vi "(백업)ATC예문V2.vi"() -> ()   [LabVIEW 2014]
doc: "ATC app"
uses:
  <vilib>/Utility/sysdir.llb/System Directory Type.ctl
panel:
  in  "정규식 5":string
  in  "정규식 4":string
  in  "?":bool
  in  "?":bool
  in  "정규식 3":string
  out "ip address":string="ip address"
  in  "탭":T1(tab)
  in  "도움말":bool
  in  "메모":string="필요한 메모를 할수 있습니다. "
  in  "SID&RadarVector. 2":string="SID&RadarVector. "
  in  "인사말":string="인사말"
  in  "관제기관":string="관제기관"
  in  "콜사인":string="콜사인\n콜사인\n콜사인"
  in  "도착공항":string="도착공항"
  in  "SID&RadarVector":string="SID&RadarVector"
  in  "비행고도":string="비행고도"
  in  "인사말2":string="인사말"
  in  "콜사인2":string="콜사인"
  in  "콜사인3":string="콜사인"
  in  "콜사인4":string="콜사인"
  in  "콜사인5":string="콜사인"
  in  "콜사인6":string="콜사인"
  in  "도착공항2":string="도착공항"
  in  "제한고도":string="제한고도"
  in  "비행고도2":string="비행고도"
  in  "D접속주파수":string="접속주파수"
  in  "스콱번호":string="스콱번호"
  in  "도착공항3":string="도착공항"
  in  "SID&RadarVector. 3":string="SID&RadarVector. "
  in  "제한고도2":string="제한고도"
  in  "비행고도3":string="비행고도"
  in  "D접속주파수2":string="접속주파수"
  in  "스콱번호2":string="스쾃번호"
  in  "콜사인7":string="콜사인"
  in  "콜사인8":string="콜사인"
  in  "관제기관":string="관제기관"
  in  "G접속주파수2":string="접속주파수"
  in  "관제기관":string="관제기관"
  in  "G접속주파수":string="접속주파수"
  in  "콜사인9":string="콜사인"
  in  "정보1":bool
  in  "도움말 2":bool
  in  "유도로 2":string="유도로"
  in  "유도로":string="유도로"
  in  "방향 2":string="방향"
  in  "방향":string="방향"
  in  "메모2":string="필요한 메모를 할수 있습니다. "
  in  "관제기관":string="관제기관"
  in  "콜사인24":string="콜사인"
  in  "T접속주파수2":string="접속주파수"
  in  "T접속주파수":string="접속주파수"
  in  "관제기관8":string="관제기관"
  in  "콜사인23":string="콜사인"
  in  "활주로9":string="활주로"
  in  "관제기관7":string="관제기관"
  in  "콜사인22":string="콜사인"
  in  "콜사인21":string="콜사인"
  in  "콜사인20":string="콜사인"
  in  "콜사인19":string="콜사인"
  in  "활주로8":string="활주로"
  in  "활주로7":string="활주로"
  in  "콜사인17":string="콜사인"
  in  "활주로6":string="활주로"
  in  "콜사인18":string="콜사인"
  in  "활주로5":string="활주로"
  in  "콜사인16":string="콜사인"
  in  "활주로4":string="활주로"
  in  "콜사인15":string="콜사인"
  in  "활주로3":string="활주로"
  in  "콜사인14":string="콜사인"
  in  "콜사인13":string="콜사인"
  in  "현재기압2":string="현재기압"
  in  "출발공항":string="출발공항"
  in  "활주로2":string="활주로"
  in  "현재기압":string="현재기압"
  in  "출발공항2":string="출발공항"
  in  "활주로1":string="활주로"
  in  "콜사인12":string="콜사인"
  in  "콜사인11":string="콜사인"
  in  "관제기관":string="관제기관"
  in  "인사3":string="인사"
  in  "정보2":bool
  in  "도움말 3":bool
  in  "콜사인34 2":string="콜사인"
  in  "관제기관 2":string="관제기관"
  in  "관제기관":string="관제기관"
  in  "관제기관":string="관제기관"
  in  "메모3":string="필요한 메모를 할수 있습니다. "
  in  "인사4":string="인사"
  in  "콜사인25":string="콜사인"
  in  "활주로10":string="활주로"
  in  "콜사인26":string="콜사인"
  in  "바람방향":string="바람방향"
  in  "풍속":string="풍속"
  in  "콜사인28":string="콜사인"
  in  "활주로13":string="활주로"
  in  "콜사인29":string="콜사인"
  in  "활주로12":string="활주로"
  in  "콜사인30":string="콜사인"
  in  "활주로14":string="활주로"
  in  "콜사인31":string="콜사인"
  in  "활주로15":string="활주로"
  in  "관제기관":string="관제기관"
  in  "콜사인32":string="콜사인"
  in  "현재고도":string="현재고도"
  in  "허가고도":string="허가고도"
  in  "콜사인33":string="콜사인"
  in  "접속주파수":string="접속주파수"
  in  "콜사인34":string="콜사인"
  in  "접속주파수2":string="접속주파수"
  in  "정보3":bool
  in  "도움말 4":bool
  in  "순항고도or이니셜고도":string="순항고도or이니셜고도"
  in  "관제기관 3":string="관제기관"
  in  "메모 4":string="필요한 메모를 할수 있습니다. "
  in  "인사5":string="인사"
  in  "관제기관":string="관제기관"
  in  "콜사인35":string="콜사인"
  in  "현재고도A":string="현재고도"
  in  "콜사인36":string="콜사인"
  in  "관제기관":string="관제기관"
  in  "허가고도4":string="허가고도"
  in  "허가고도5":string="허가고도"
  in  "콜사인37":string="콜사인"
  in  "콜사인38":string="콜사인"
  in  "허가고도6":string="허가고도"
  in  "허가고도7":string="허가고도"
  in  "콜사인39":string="콜사인"
  in  "콜사인40":string="콜사인"
  in  "관제기관":string="관제기관"
  in  "A접속주파수":string="접속주파수"
  in  "관제기관14":string="관제기관"
  in  "A접속주파수2":string="접속주파수"
  in  "콜사인41":string="콜사인"
  in  "정보4":bool
  in  "콜사인38 2":string="콜사인"
  in  "관제기관 4":string="관제기관"
  in  "허가고도6 2":string="허가고도"
  in  "허가고도6 3":string="허가고도"
  in  "콜사인39 2":string="콜사인"
  in  "메모5":string="필요한 메모를 할수 있습니다. "
  in  "도움말 5":bool
  in  "정보5":bool
  in  "인사말 2":string="인사말"
  in  "허가고도 2":string="허가고도"
  in  "지점":string="지점"
  in  "허가고도7 2":string="허가고도"
  in  "콜사인38 3":string="콜사인"
  in  "콜사인39 3":string="콜사인"
  in  "허가고도7 3":string="허가고도"
  in  "지점 2":string="지점"
  in  "메모6":string="필요한 메모를 할수 있습니다. "
  in  "도움말 6":bool
  in  "관제기관":string="관제기관"
  in  "콜사인46":string="콜사인"
  in  "날시정보":string="날시정보"
  in  "고도":string="고도"
  in  "콜사인47":string="콜사인"
  in  "관제기관":string="관제기관"
  in  "L활주로":string="활주로"
  in  "도착공항4":string="도착공항"
  in  "현재기압":string="현재기압"
  in  "콜사인48":string="콜사인"
  in  "관제기관5":string="관제기관"
  in  "L활주로":string="활주로"
  in  "도착공항5":string="도착공항"
  in  "현재기압":string="현재기압"
  in  "콜사인49":string="콜사인"
  in  "고도":string="고도"
  in  "콜사인50":string="콜사인"
  in  "고도":string="고도"
  in  "콜사인51":string="콜사인"
  in  "고도":string="고도"
  in  "고도":string="고도"
  in  "콜사인52":string="콜사인"
  in  "콜사인53":string="콜사인"
  in  "관제기관":string="관제기관"
  in  "풍속":string="풍속"
  in  "바람방향":string="바람방향"
  in  "L활주로3":string="활주로"
  in  "콜사인54":string="콜사인"
  in  "L활주로":string="활주로"
  in  "콜사인55":string="콜사인"
  in  "관제기관":string="관제기관"
  in  "L활주로":string="활주로"
  in  "ILS":string="주파수(ils)"
  in  "콜사인56":string="콜사인"
  in  "L활주로6":string="활주로"
  in  "ILS2":string="주파수(ils)"
  in  "콜사인57":string="콜사인"
  in  "T관제기관":string="관제기관"
  in  "T접속주파수":string="접속주파수"
  in  "콜사인58":string="콜사인"
  in  "콜사인59":string="콜사인"
  in  "관제기관":string="관제기관"
  in  "T접속주파수":string="접속주파수"
  in  "정보6":bool
  in  "메모7":string="필요한 메모를 할수 있습니다. "
  in  "도움말 7":bool
  in  "바람방향":string="바람방향"
  in  "관제기관":string="관제기관"
  in  "콜사인60":string="콜사인"
  in  "L활주로7":string="활주로"
  in  "콜사인61":string="콜사인"
  in  "풍속":string="풍속"
  in  "콜사인62":string="콜사인"
  in  "L활주로":string="활주로"
  in  "L활주로":string="활주로"
  in  "관제기관":string="관제기관"
  in  "콜사인63":string="콜사인"
  in  "관제기관3":string="관제기관"
  in  "콜사인64":string="콜사인"
  in  "L활주로":string="활주로"
  in  "G관제기관":string="관제기관"
  in  "G접속주파수":string="접속주파수"
  in  "콜사인65":string="콜사인"
  in  "관제기관":string="관제기관"
  in  "G접속주파수":string="접속주파수"
  in  "정보7":bool
  in  "콜사인70":string="콜사인"
  in  "C활주로3":string="활주로"
  in  "C활주로2":string="활주로"
  in  "관제기관3 2":string="관제기관"
  in  "C활주로":string="활주로"
  in  "콜사인69":string="콜사인"
  in  "관제기관2":string="관제기관"
  in  "메모8":string="필요한 메모를 할수 있습니다. "
  in  "도움말 8":bool
  in  "관제기관":string="관제기관"
  in  "콜사인66":string="콜사인"
  in  "콜사인67":string="콜사인"
  in  "게이트번호":string="게이트번호"
  in  "THEN":string="then"
  in  "콜사인68":string="콜사인"
  in  "게이트번호2":string="게이트번호"
  in  "THEN2":string="then"
  in  "콜사인10":string="콜사인"
  in  "관제기관4":string="관제기관"
  in  "콜사인71":string="콜사인"
  in  "콜사인72":string="콜사인"
  in  "정보8":bool
  # "ver.Beta.2.2.0"
  # "~"
  # "Good"
  # "Clearance Delivery"
  # "Pilot"
  # "at FL"
  # "Request IFR Clearance to"
  # "Airport via"
  # "~"
  # "Good"
  # "Controller"
  # ",  Clearance  Delivery, standby."
  # "Pilot"
  # "Stand by,"
  # "Controller"
  # "Delivery 또는 Delivery, Are you ready to copy?"
  # "Pilot"
  # "Go Ahead 또는 Ready to copy"
  # "Airport via"
  # ", Cleared to"
  # "Controller"
  # "ft expect FL"
  # "then as filed. Climb and Maintain"
  # "Departure Frequency"
  # "Read back."
  # "Squawk"
  # "Pilot"
  # "Airport via"
  # "Cleared to"
  # ","
  # "then as filed."
  # "Climb and Maintain"
  # "ft expect FL"
  # "Departure Frequency"
  # "and  Squawk"
  # "Controller"
  # ", Read back is corrent contact"
  # "Ground"
  # "bye bye~."
  # "Pilot"
  # "Roger, contact"
  # ", bye bye~"
  # "ver.Beta.2.2.0"
  # "Pilot"
  # "~"
  # "Good"
  # "ready for push back and Engine Start."
  # ","
  # ", Rwy"
  # "Push Back and Engine Start Approved, heading to"
  # "Controller"
  # ","
  # "QNH"
  # "Read Back."
  # "Pilot"
  # "Roger\nPush Back and Engine Start Approved, heading to"
  # ", Rwy"
  # "QNH"
  # "Ready for taxi to the Rwy"
  # ","
  # "Pilot"
  # "- Push back 완료 후 -"
  # ", Ready for Taxi to Rwy"
  # "Controller"
  # ", taxi to"
  # "via taxiway"
  # ", Roger"
  # "Pilot"
  # "via taxiway"
  # "Taxi to"
  # "- 활주로를 건널 상황일 때 -"
  # "Pilot"
  # "Request Cross Rwy"
  # "Controller"
  # ", cleared Cross Rwy"
  # "Pilot"
  # "cleared Cross Rwy"
  # "Controller"
  # "Squawk Mode C."
  # "Pilot"
  # ", Roger squawk mode 'C'"
  # "------------------------ 홀딩 포인트 도착 후 ----------------------------------"
  # "hold short of Rwy"
  # ","
  # "Controller"
  # "Roger,"
  # "contact"
  # "Tower"
  # "bye bye~"
  # "Pilot"
  # "Contact"
  # "ver.Beta.2.2.0"
  # "Pilot"
  # "Good"
  # "~"
  # ",  hold short Rwy"
  # ", Ready for Departure"
  # "(곧바로 이륙허가)"
  # "Controller"
  # ", wind"
  # "knot, cleared for take off."
  # "at"
  # "(활주로 정렬대기)"
  # "Controller"
  # "Line up and wait Rwy"
  # "Pilot"
  # "Line up and wait Rwy"
  # "Roger,"
  # "(홀딩 포인트에서 대기)"
  # "Controller"
  # ", Hold short rwy"
  # ","
  # "Pilot"
  # "Hold short of Rwy"
  # "Roger,"
  # "- 이 륙 후 -"
  # "ft."
  # "Pilot"
  # "Airborn Passing"
  # "ft, Climbing"
  # ","
  # "Controller"
  # ", contact"
  # "Departure,"
  # "bye bye~"
  # "Pilot"
  # ", Roger"
  # "Contact"
  # "Departure,"
  # "bye bye~"
  # "ver.Beta.2.2.0"
  # "Good"
  # "~"
  # "Pilot"
  # "Passing"
  # "expect"
  # "with (SID)."
  # ","
  # ","
  # "Controller"
  # "Departure, Radar Contact, Climb via (SID) to"
  # ","
  # "."
  # "Pilot"
  # "Roger, Climb via"
  # ","
  # "-고도제한 해제시-"
  # "Controller"
  # "Departure, Radar Contact, Climb via (SID) to"
  # ", Cancel Level Restrictions."
  # "Pilot"
  # "Roger, Climb via (SID) to"
  # ", Cancel Level Restrictions,"
  # "-속도제한 해제시-"
  # "Controller"
  # "Departure, Radar Contact, Climb via (SID) to"
  # ", Cancel Speed Restrictions."
  # "Pilot"
  # "Roger, Climb via (SID) to"
  # ", Cancel Speed Restrictions,"
  # "Controller"
  # "Control,"
  # ", bye bye."
  # ", You are leaving my airspace, Contact"
  # "Pilot"
  # "Contact"
  # "G'day"
  # "Control,"
  # ","
  # "ver.Beta.2.2.0"
  # "Pilot"
  # "Good"
  # "Decend and maintain FL"
  # "with (SID)."
  # "-하강 발부-"
  # "Controller"
  # "by"
  # ", Descend and Maintain"
  # "Pilot"
  # "Descend and Maintain"
  # "by"
  # "Pilot"
  # "ver.Beta.2.2.0"
  # ","
  # "FL"
  # "with information"
  # ","
  # ", Expect vector to ILS Rwy"
  # "approach"
  # "Controller"
  # "QNH"
  # "Roger,"
  # "Pilot"
  # ", Expect vector to ILS Rwy"
  # "final approach"
  # "QNH"
  # "Controller"
  # ", Decend and maintain FL"
  # "Pilot"
  # "Decend and maintain FL"
  # "Roger,"
  # "Controller"
  # ", Decend and maintain"
  # "ft"
  # "Pilot"
  # "Roger"
  # "Decend and maintain"
  # "ft"
  # "Controller"
  # ","
  # "for landing"
  # "wind"
  # "knots active Rwy"
  # "at"
  # "Pilot"
  # "Roger,"
  # "Rwy"
  # "for landing"
  # "Controller"
  # ","
  # "approach use Rwy"
  # "ILS"
  # "Roger,"
  # "Pilot"
  # "Use Rwy"
  # "ILS"
  # "- 정 렬 후 -"
  # "Pilot"
  # "Approach,"
  # ", Established on Localizer."
  # "Controller"
  # "Tower,"
  # "Good day,"
  # "Roger, Contact"
  # "Pilot"
  # "Contact"
  # "Tower"
  # "Good day,"
  # "ver.Beta.2.2.0"
  # "Pilot"
  # ","
  # "Inbound Approaching Rwy"
  # "Controller"
  # ", Wind"
  # "at"
  # "knots Rwy"
  # ", Cleared to land"
  # "Pilot"
  # "Rwy"
  # "Cleared to land"
  # "Pilot"
  # ","
  # "- 착 륙 후 -"
  # ","
  # "Pilot"
  # "Touch down with Rwy"
  # "Controller"
  # "Roger, change squawk mode Standby and contact"
  # "bye bye~"
  # "ground"
  # "Pilot"
  # ", Roger"
  # "bye bye~"
  # "Change squawk mode standby and contact"
  # "- 활주로를 건널 상황일 때 -"
  # "Pilot"
  # ","
  # "Request Cross Rwy"
  # "Controller"
  # ", Cross Rwy"
  # "approved."
  # "Pilot"
  # "Cross Rwy"
  # "approved"
  # "ver.Beta.2.2.0"
  # ","
  # "Pilot"
  # "Ready to taxi to the Gate"
  # "Controller"
  # ", taxi to the gate"
  # "via taxi way"
  # "Roger,"
  # "Pilot"
  # "taxi to the gate"
  # "via taxi way"
  # "- 게이트 도착 후 -"
  # "Pilot"
  # "at Gate and Engine Shut down."
  # "Thank you for your ATC service."
  # "Controller"
  # ", at the gate and Engine Shut down, Thank you ~~"
  # "Pilot"
  # "Have a nice day,"
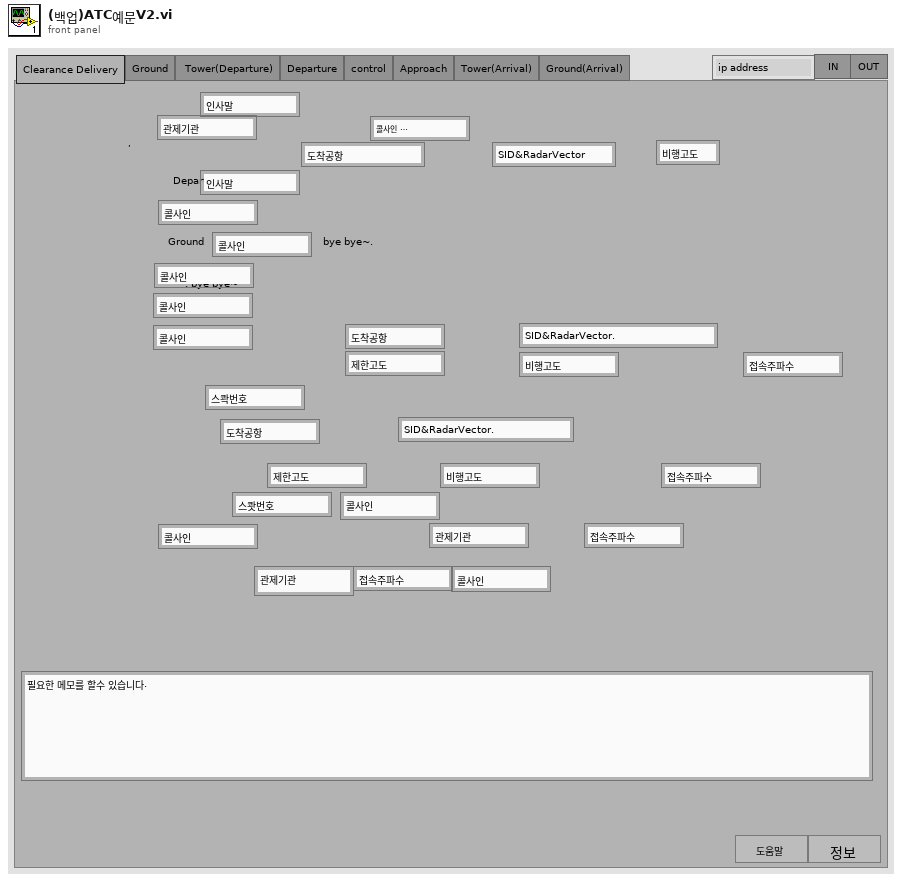
[diagram p1: front panel]
types:
  T1 = enum32{"Clearance Delivery", "Ground", " Tower(Departure)", "Departure", "control", "Approach", "Tower(Arrival)", "Ground(Arrival)"}
  T2 = enum16{"open", "replace", "create", "open or create", "replace or create", "replace or create with confirmation"}
  T3 = typedef "System Directory Type.ctl" = i32
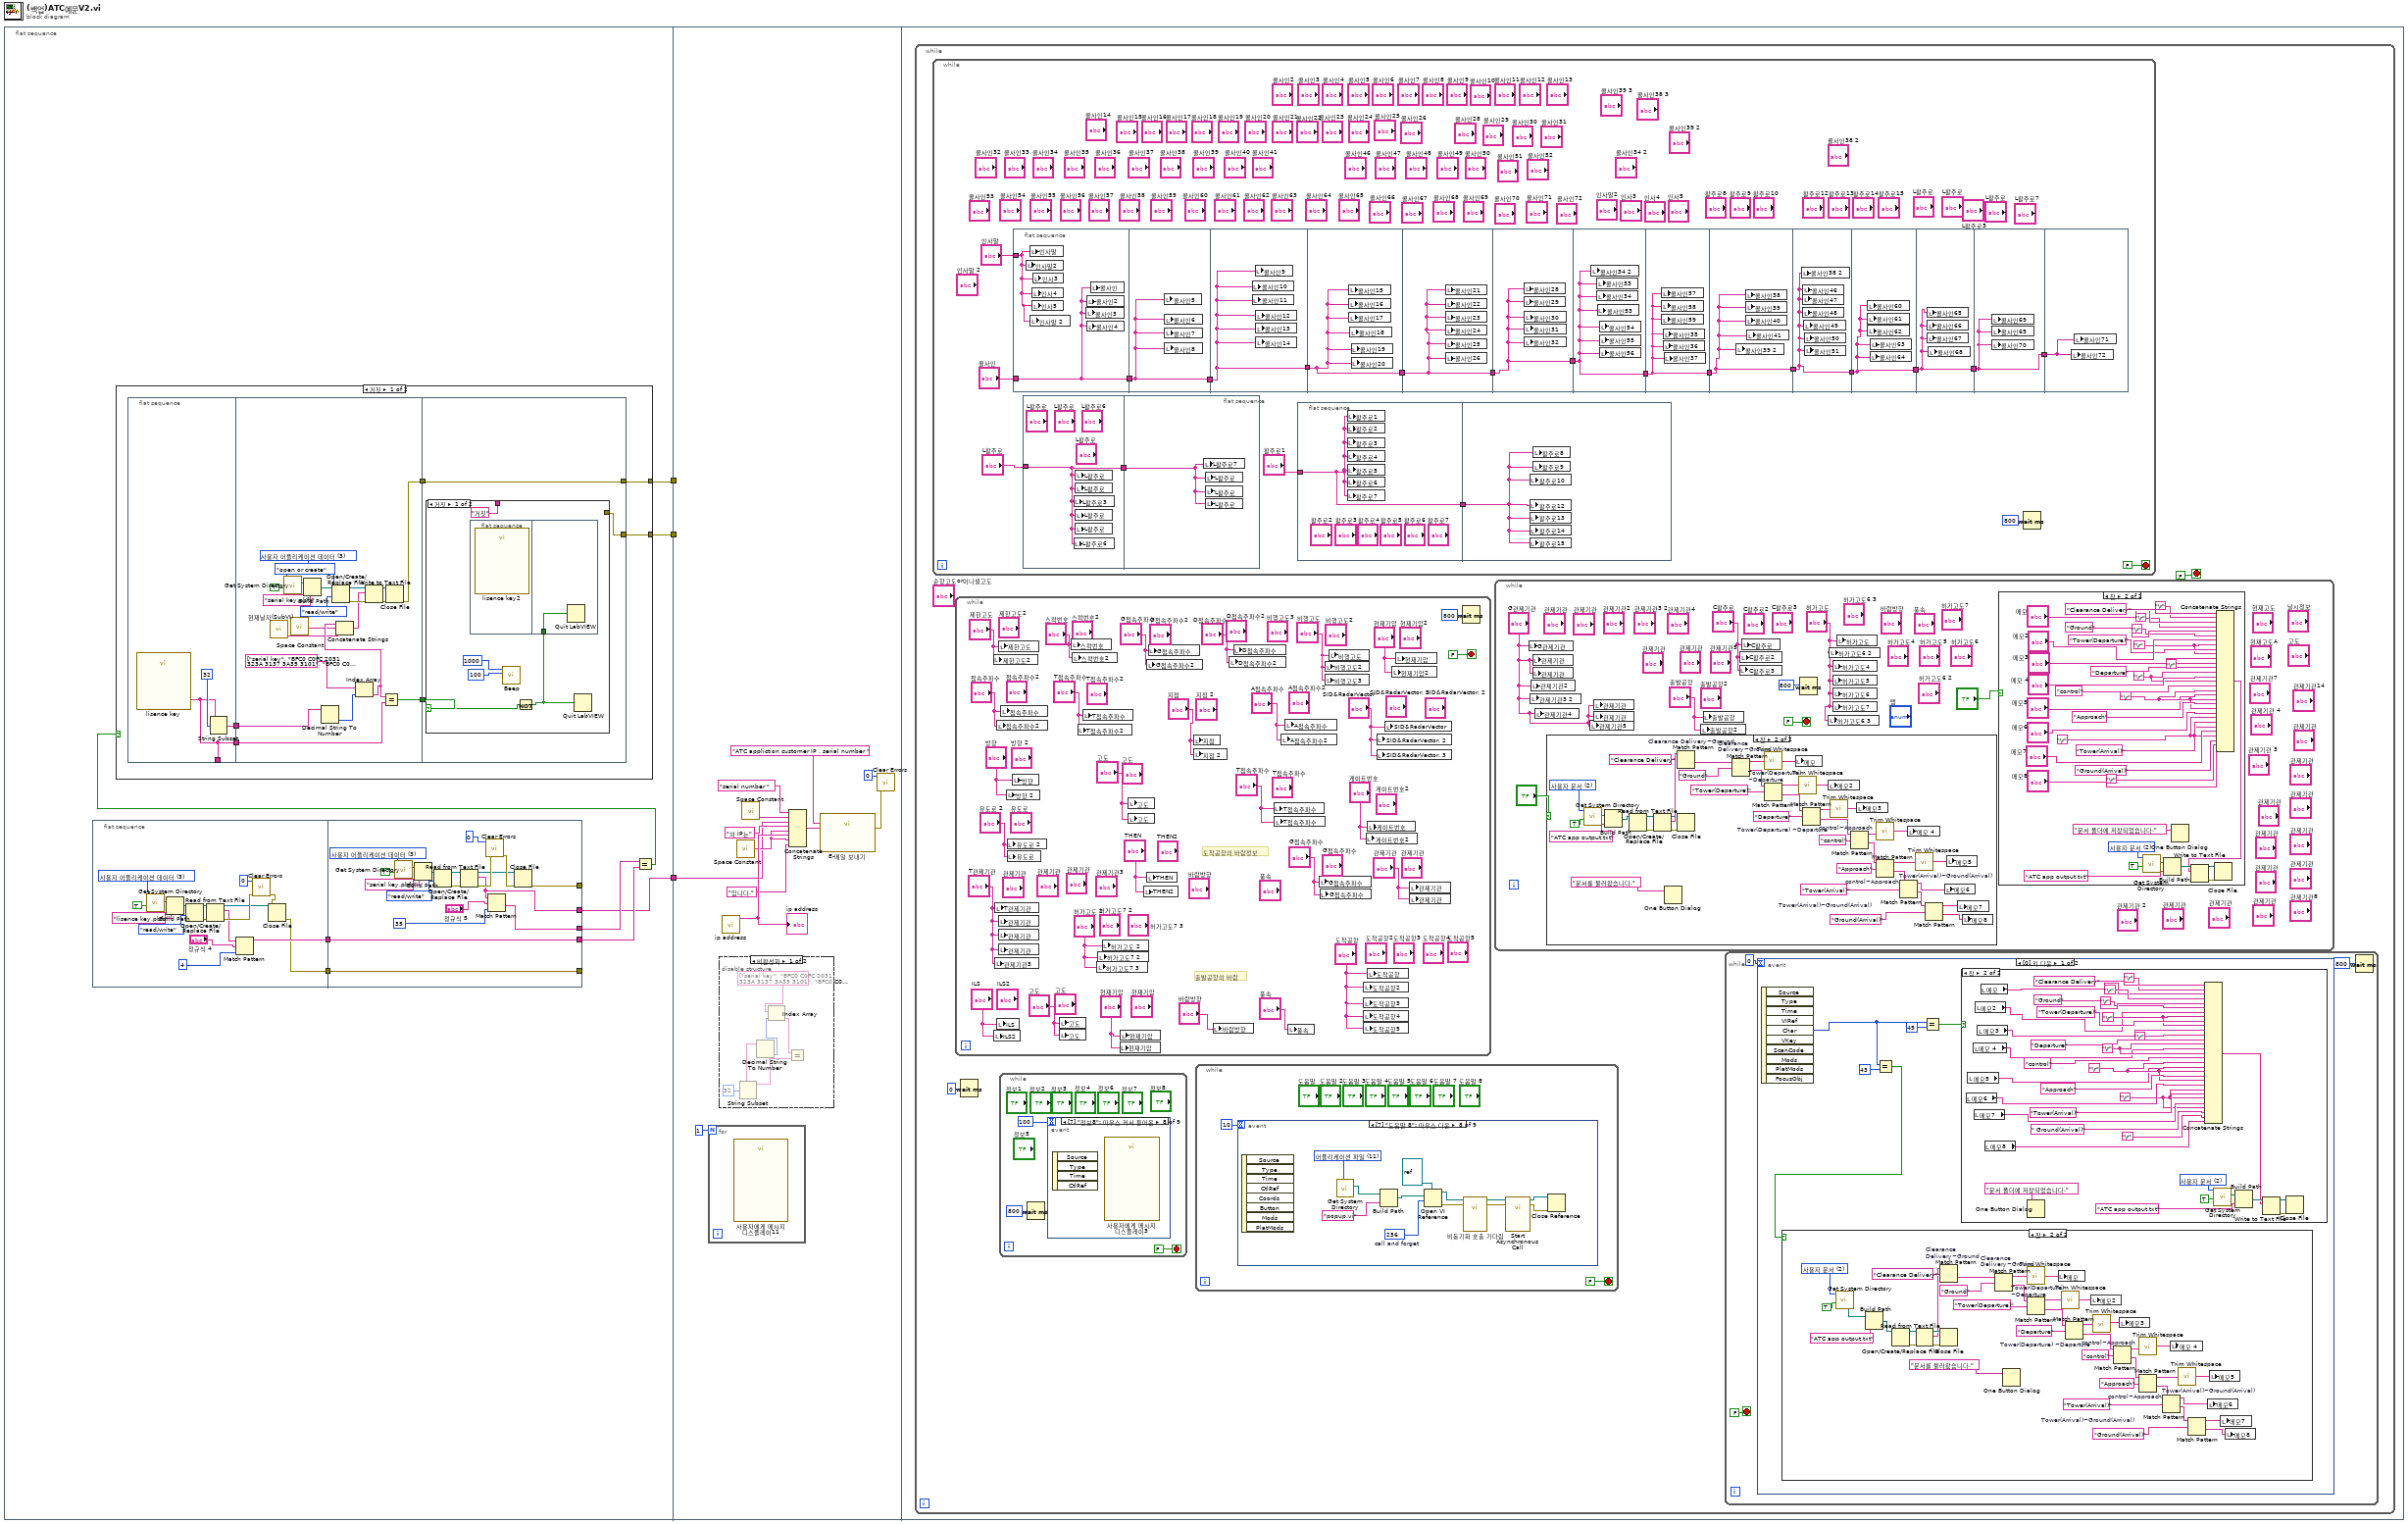
[diagram p0: block diagram]
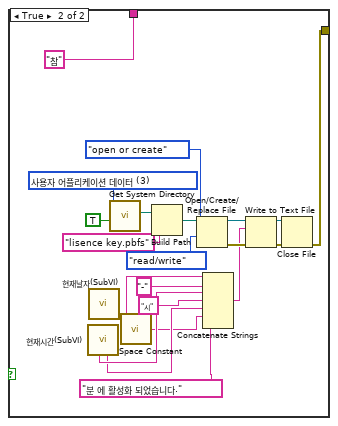
[diagram p2: hidden frame]
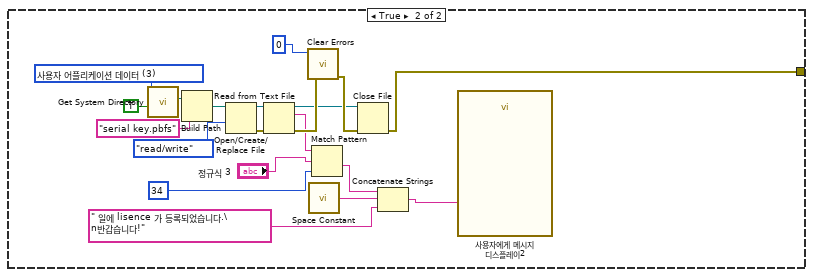
[diagram p3: hidden frame]
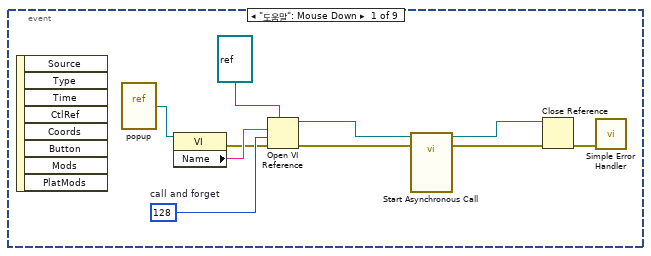
[diagram p5: hidden frame]
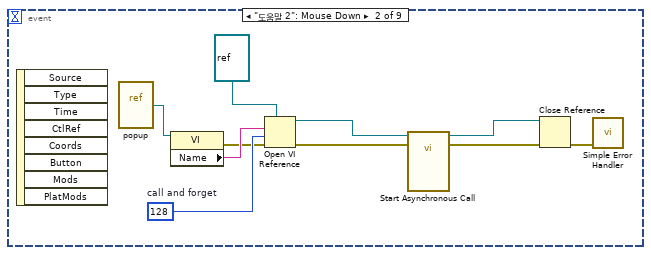
[diagram p6: hidden frame]
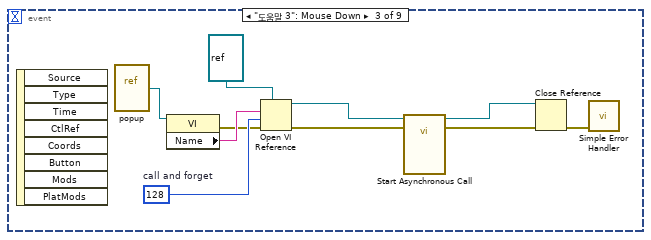
[diagram p7: hidden frame]
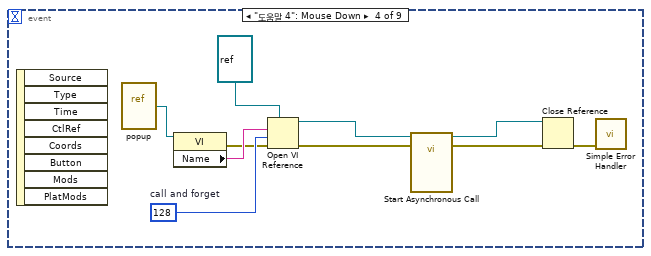
[diagram p8: hidden frame]
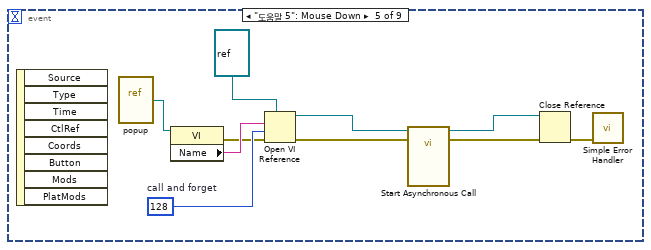
[diagram p9: hidden frame]
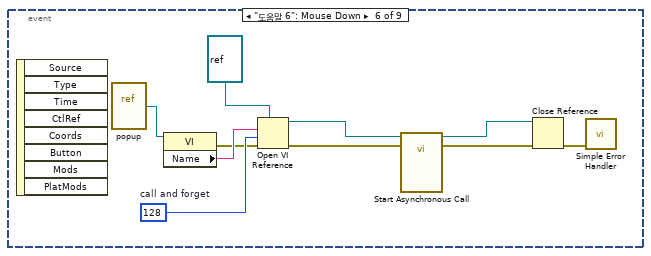
[diagram p10: hidden frame]
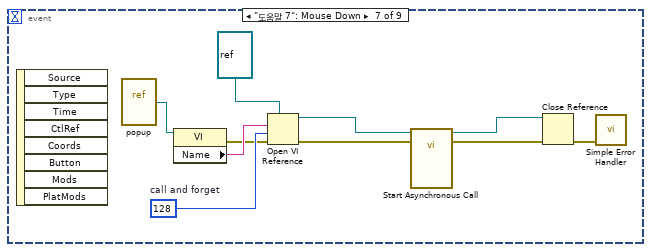
[diagram p11: hidden frame]
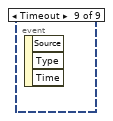
[diagram p12: hidden frame]
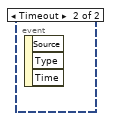
[diagram p15: hidden frame]
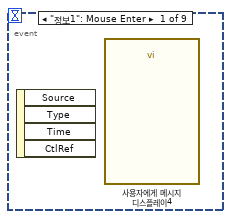
[diagram p16: hidden frame]
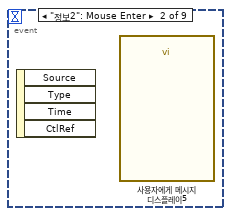
[diagram p17: hidden frame]
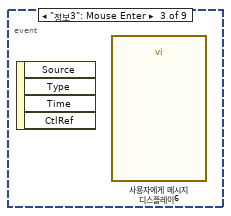
[diagram p18: hidden frame]
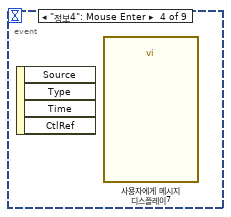
[diagram p19: hidden frame]
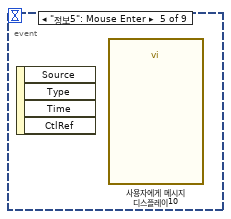
[diagram p20: hidden frame]
diagram:
  n1 = flat-sequence {
    tunnel: [w4] -> w3
    tunnel: [w11] -> w2
    tunnel: [w10] -> w1
    tunnel: w3 -> [w128]
    tunnel: w2 -> [_]
    tunnel: w1 -> [_]
    frame #0 {
      n2 = flat-sequence {
        tunnel: [w13] -> w9
        tunnel: [w12] -> w8
        tunnel: [w35] -> w6
        tunnel: w9 -> [w35]
        tunnel: [w33] -> w7
        tunnel: [w29] -> w4
        tunnel: [w31] -> _
        tunnel: w8 -> [w31]
        tunnel: [w30] -> _
        frame #0 {
          w18 = T3 3 items=["사용자 홈"=0, "사용자 데스크탑"=1, "사용자 문서"=2, "사용자 어플리케이션 데이터"=3, "사용자 환경"=4, "사용자 임시"=5, "퍼블릭 문서"=6, "퍼블릭 어플리케이션 데이터"=7, "퍼블릭 환경"=8, "퍼블릭 캐시"=13, "시스템 코어 라이브러리"=9, "시스템 설치된 라이브러리"=10, "어플리케이션 파일"=11, "부팅 볼륨 루트"=12] ("system directory type")
          n3 = call <vilib>:"Get System Directory.vi"("create directory if not found? (F)"=TRUE, "system directory type"=w18) -> ("system directory"=w17:path)  [unwired: 9 in]
          n4 = Build Path(base path=w17, name or relative path="lisence key.pbfs" ("이름 또는 상대 경로")) -> (appended path=w16:path)
          n5 = Open/Create/Replace File(file path (use dialog)=w16, access (0:read/write)=enum16{"read/write", "read-only", "write-only"}."read/write" ("접근(0:읽기/쓰기)")) -> (refnum out=w22:refnum<file>, error out=w21:errorcluster)  [unwired: 4 in, 1 out]
          n6 = Read from Text File(file (use dialog)=w22, error in=w21) -> (refnum out=w23:refnum<file>, text=w24:string, error out=w26:errorcluster)  [unwired: 2 in, 1 out]
          n7 = Match Pattern(string=w24, regular expression="정규식 4", offset (0)=4 ("오프셋(0) 2")) -> (before substring=w13:string)  [unwired: 3 out]
          n8 = call <vilib>:"Clear Errors.vi"("error in (no error)"=w26, "specific error code to clear (0: all)"=0) -> ("error out"=w27:errorcluster)  [unwired: 4 in, 1 out]
          n9 = Close File(refnum=w23, error in=w27) -> (error out=w12:errorcluster)  [unwired: 1 out]
        }
        frame #1 {
          w41 = T3 3 items=["사용자 홈"=0, "사용자 데스크탑"=1, "사용자 문서"=2, "사용자 어플리케이션 데이터"=3, "사용자 환경"=4, "사용자 임시"=5, "퍼블릭 문서"=6, "퍼블릭 어플리케이션 데이터"=7, "퍼블릭 환경"=8, "퍼블릭 캐시"=13, "시스템 코어 라이브러리"=9, "시스템 설치된 라이브러리"=10, "어플리케이션 파일"=11, "부팅 볼륨 루트"=12] ("system directory type")
          n10 = call <vilib>:"Get System Directory.vi"("create directory if not found? (F)"=TRUE, "system directory type"=w41) -> ("system directory"=w42:path)  [unwired: 9 in]
          n11 = Build Path(base path=w42, name or relative path="serial key.pbfs" ("이름 또는 상대 경로")) -> (appended path=w43:path)
          n12 = Open/Create/Replace File(file path (use dialog)=w43, access (0:read/write)=enum16{"read/write", "read-only", "write-only"}."read/write" ("접근(0:읽기/쓰기)")) -> (refnum out=w37:refnum<file>, error out=w38:errorcluster)  [unwired: 4 in, 1 out]
          n13 = Read from Text File(file (use dialog)=w37, error in=w38) -> (refnum out=w36:refnum<file>, text=w29:string, error out=w45:errorcluster)  [unwired: 2 in, 1 out]
          n14 = call <vilib>:"Clear Errors.vi"("error in (no error)"=w45, "specific error code to clear (0: all)"=0) -> ("error out"=w46:errorcluster)  [unwired: 4 in, 1 out]
          n15 = Match Pattern(string=w29, regular expression="정규식 5", offset (0)=35 ("오프셋(0)")) -> (after substring=w33:string)  [unwired: 3 out]
          n16 = Close File(refnum=w36, error in=w46) -> (error out=w30:errorcluster)  [unwired: 1 out]
        }
      }
      n17 = Equal?(x=w7, y=w6) -> (x = y?=w5:bool)
      n18 = case shown="거짓" w5 {
        tunnel: [w49 w108] -> w10
        tunnel: [w48 _] -> w11
        frame False {
          n19 = flat-sequence {
            tunnel: [w55] -> w53
            tunnel: [w54] -> w52
            tunnel: [w54] -> _
            tunnel: w53 -> [w77]
            tunnel: [w74] -> w51
            tunnel: w52 -> [w75]
            tunnel: [w58] -> w50
            tunnel: w51 -> [w80]
            tunnel: [w79] -> w49
            tunnel: w50 -> [w78]
            tunnel: [w78] -> w48
            frame #0 {
              n20 = call "lisence key"() -> ("lisence key"=w54:string)  [unwired: 17 in, 2 out]
              n21 = String Subset(string=w54, offset (0)=32 ("오프셋(0)")) -> (substring=w55:string)  [unwired: 1 in]
            }
            frame #1 {
              w67 = T3 3 items=["사용자 홈"=0, "사용자 데스크탑"=1, "사용자 문서"=2, "사용자 어플리케이션 데이터"=3, "사용자 환경"=4, "사용자 임시"=5, "퍼블릭 문서"=6, "퍼블릭 어플리케이션 데이터"=7, "퍼블릭 환경"=8, "퍼블릭 캐시"=13, "시스템 코어 라이브러리"=9, "시스템 설치된 라이브러리"=10, "어플리케이션 파일"=11, "부팅 볼륨 루트"=12] ("system directory type")
              n22 = call "현재날자(SubVI).vi"() -> ("월,일 을 문자열로"=w62:string)  [unwired: 5 in, 6 out]
              n23 = call <vilib>:"Get System Directory.vi"("create directory if not found? (F)"=TRUE, "system directory type"=w67) -> ("system directory"=w66:path)  [unwired: 9 in]
              n24 = call <vilib>:"Space Constant.vi"() -> ("String"=w61:string)
              n25 = Build Path(base path=w66, name or relative path="serial key.pbfs" ("이름 또는 상대 경로")) -> (appended path=w65:path)
              n26 = Decimal String To Number(string=w77) -> (number=w76:i32)  [unwired: 2 in, 1 out]
              n27 = Open/Create/Replace File(file path (use dialog)=w65, operation (0:open)=T2."open or create" ("동작(0:open)"), access (0:read/write)=enum16{"read/write", "read-only", "write-only"}."read/write" ("접근(0:읽기/쓰기)")) -> (refnum out=w73:refnum<file>, error out=w72:errorcluster)  [unwired: 3 in, 1 out]
              n28 = Index Array(array=string[] ["serial key", "BFC0 C0FC 2031 323A 3137 3A35 3101", "BFC0 C0FC 2031 323A 3138 3A30 3902", "BFC0 C0FC 2031 323A 3139 3A30 3903", "BFC0 C0FC 2031 323A 3230 3A30 3904", "BFC0 C0FC 2031 323A 3231 3A30 3905", "BFC0 C0FC 2031 323A 3232 3A30 3906", "BFC0 C0FC 2031 323A 3233 3A30 3907", "BFC0 C0FC 2031 323A 3234 3A30 3908", "BFC0 C0FC 2031 323A 3235 3A30 3909", "BFC0 C0FC 2031 323A 3236 3A30 3910", "BFC0 C0FC 2031 323A 3237 3A30 3911", "BFC0 C0FC 2031 323A 3238 3A30 3912", "BFC0 C0FC 2031 323A 3239 3A30 3913", "BFC0 C0FC 2031 323A 3036 3A33 3214", "BFC0 C0FC 2031 323A 3037 3A33 3215", "BFC0 C0FC 2031 323A 3038 3A33 3216", "BFC0 C0FC 2031 323A 3038 3A33 3217", "BFC0 C0FC 2031 323A 3039 3A33 3218", "BFC0 C0FC 2031 323A 3039 3A35 3019", "BFC0 C0FC 2031 323A 3130 3A35 3020", "BFC0 C0FC 2031 323A 3131 3A35 3121", "BFC0 C8C4 2031 313A 3536 3A33 3222", "BFC0 C8C4 2031 313A 3537 3A33 3223", "BFC0 C8C4 2031 313A 3538 3A33 3224", "BFC0 C8C4 2031 313A 3539 3A33 3225", "BFC0 C0FC 2031 323A 3030 3A33 3226", "BFC0 C0FC 2031 323A 3031 3A33 3227", "BFC0 C0FC 2031 323A 3032 3A33 3228", "BFC0 C0FC 2031 323A 3033 3A33 3229", "BFC0 C0FC 2031 323A 3034 3A33 3230", "BFC0 C0FC 2031 323A 3035 3A33 3231", "BFC0 C0FC 2031 323A 3036 3A33 3232", "BFC0 C0FC 2031 323A 3037 3A33 3233", "BFC0 C0FC 2031 323A 3038 3A33 3234", "BFC0 C0FC 2033 3A34 373A 3031 0035 ", "BFC0 C0FC 2033 3A34 383A 3234 0036", "BFC0 C0FC 2033 3A34 393A 3132 0037", "BFC0 C0FC 2033 3A35 303A 3534 0038", "BFC0 C0FC 2033 3A35 313A 3231 0039 ", "BFC0 C0FC 2033 3A35 323A 3333 0040 ", "BFC0 C0FC 2033 3A35 333A 3030 0041", "BFC0 C0FC 2033 3A35 343A 3432 0042", "BFC0 C0FC 2033 3A35 353A 3431 0043", "BFC0 C0FC 2033 3A35 363A 3131 0044", "BFC0 C0FC 2033 3A35 373A 3239 0045", "BFC0 C0FC 2033 3A35 383A 3539 0046", "BFC0 C0FC 2033 3A35 393A 3533 0047", "BFC0 C0FC 2034 3A30 303A 3430 0048 "] ("출력 배열"), index=w76) -> (element=w63:string)
              n29 = Concatenate Strings(w63, w61, w62) -> (w64:string)
              n30 = Write to Text File(file (use dialog)=w73, text=w64, error in=w72) -> (refnum out=w70:refnum<file>, error out=w71:errorcluster)  [unwired: 1 in, 1 out]
              n31 = Equal?(x=w63, y=w75) -> (x = y?=w74:bool)
              n32 = Close File(refnum=w70, error in=w71) -> (error out=w58:errorcluster)  [unwired: 1 out]
            }
            frame #2 {
              n33 = case shown="거짓" w80 {
                selector: w80 -> [w83 _]
                tunnel: ["거짓" "참"] -> _
                tunnel: [_ w87] -> w79
                frame False {
                  n34 = flat-sequence {
                    tunnel: w84 -> [w86]
                    frame #0 {
                      n35 = call "lisence key2"() -> ()  [unwired: 10 in, 2 out]
                    }
                    frame #1 {
                      n36 = Quit LabVIEW(quit? (T)=w86) -> ()
                    }
                  }
                  n37 = call <vilib>:"Beep.vi"("duration (msec)"=u32 100, "frequency (Hz)"=u32 1000) -> ()  [unwired: 10 in]
                  n38 = Not(x=w83) -> (.not. x?=w84:bool)
                  n39 = Quit LabVIEW(quit? (T)=w84) -> ()
                }
                frame True {
                  w103 = T3 3 items=["사용자 홈"=0, "사용자 데스크탑"=1, "사용자 문서"=2, "사용자 어플리케이션 데이터"=3, "사용자 환경"=4, "사용자 임시"=5, "퍼블릭 문서"=6, "퍼블릭 어플리케이션 데이터"=7, "퍼블릭 환경"=8, "퍼블릭 캐시"=13, "시스템 코어 라이브러리"=9, "시스템 설치된 라이브러리"=10, "어플리케이션 파일"=11, "부팅 볼륨 루트"=12] ("system directory type")
                  n40 = call "현재시간(SubVI).vi"() -> ("분 문자열"=w92:string, "시 문자열"=w94:string)  [unwired: 3 in, 7 out]
                  n41 = call "현재날자(SubVI).vi"() -> ("월,일 을 문자열로"=w96:string)  [unwired: 5 in, 6 out]
                  n42 = call <vilib>:"Get System Directory.vi"("create directory if not found? (F)"=TRUE, "system directory type"=w103) -> ("system directory"=w104:path)  [unwired: 9 in]
                  n43 = call <vilib>:"Space Constant.vi"() -> ("String"=w91:string)
                  n44 = Build Path(base path=w104, name or relative path="lisence key.pbfs" ("이름 또는 상대 경로")) -> (appended path=w105:path)
                  n45 = Open/Create/Replace File(file path (use dialog)=w105, operation (0:open)=T2."open or create" ("동작(0:open)"), access (0:read/write)=enum16{"read/write", "read-only", "write-only"}."read/write" ("접근(0:읽기/쓰기)")) -> (refnum out=w101:refnum<file>, error out=w99:errorcluster)  [unwired: 3 in, 1 out]
                  n46 = Concatenate Strings(w96, "-", w94, "시", w92, w91, "분 에 활성화 되었습니다.") -> (w97:string)
                  n47 = Write to Text File(file (use dialog)=w101, text=w97, error in=w99) -> (refnum out=w102:refnum<file>, error out=w98:errorcluster)  [unwired: 1 in, 1 out]
                  n48 = Close File(refnum=w102, error in=w98) -> (error out=w87:errorcluster)  [unwired: 1 out]
                }
              }
            }
          }
        }
        frame True {
          w121 = T3 3 items=["사용자 홈"=0, "사용자 데스크탑"=1, "사용자 문서"=2, "사용자 어플리케이션 데이터"=3, "사용자 환경"=4, "사용자 임시"=5, "퍼블릭 문서"=6, "퍼블릭 어플리케이션 데이터"=7, "퍼블릭 환경"=8, "퍼블릭 캐시"=13, "시스템 코어 라이브러리"=9, "시스템 설치된 라이브러리"=10, "어플리케이션 파일"=11, "부팅 볼륨 루트"=12] ("system directory type")
          n49 = call <vilib>:"Get System Directory.vi"("create directory if not found? (F)"=TRUE, "system directory type"=w121) -> ("system directory"=w122:path)  [unwired: 9 in]
          n50 = Build Path(base path=w122, name or relative path="serial key.pbfs" ("이름 또는 상대 경로")) -> (appended path=w123:path)
          n51 = Open/Create/Replace File(file path (use dialog)=w123, access (0:read/write)=enum16{"read/write", "read-only", "write-only"}."read/write" ("접근(0:읽기/쓰기)")) -> (refnum out=w117:refnum<file>, error out=w118:errorcluster)  [unwired: 4 in, 1 out]
          n52 = Read from Text File(file (use dialog)=w117, error in=w118) -> (refnum out=w116:refnum<file>, text=w124:string, error out=w126:errorcluster)  [unwired: 2 in, 1 out]
          n53 = call <vilib>:"Clear Errors.vi"("error in (no error)"=w126, "specific error code to clear (0: all)"=0) -> ("error out"=w127:errorcluster)  [unwired: 4 in, 1 out]
          n54 = call <vilib>:"Space Constant.vi"() -> ("String"=w110:string)
          n55 = Match Pattern(string=w124, regular expression="정규식 3", offset (0)=34 ("오프셋(0)")) -> (after substring=w113:string)  [unwired: 3 out]
          n56 = Close File(refnum=w116, error in=w127) -> (error out=w108:errorcluster)  [unwired: 1 out]
          n57 = Concatenate Strings(w113, w110, " 일에 lisence 가 등록되었습니다.\n반갑습니다!" ("Message")) -> (w112:string)
          n58 = call "사용자에게 메시지 디스플레이2"("Message"=w112) -> ()  [unwired: 9 in, 2 out]
        }
      }
    }
    frame #1 {
      n59 = for {
        N: 1 -> [_]
        n60 = call "사용자에게 메시지 디스플레이11"() -> ()  [unwired: 10 in, 2 out]
      }
      n61 = disable-structure shown="비활성화" {
        frame Disabled {
          n62 = String Subset(string=w140, offset (0)=32 ("오프셋(0)")) -> (substring=w143:string)  [unwired: 1 in]
          n63 = Decimal String To Number(string=w143) -> (number=w142:i32)  [unwired: 2 in, 1 out]
          n64 = Index Array(array=string[] ["serial key", "BFC0 C0FC 2031 323A 3137 3A35 3101", "BFC0 C0FC 2031 323A 3138 3A30 3902", "BFC0 C0FC 2031 323A 3139 3A30 3903", "BFC0 C0FC 2031 323A 3230 3A30 3904", "BFC0 C0FC 2031 323A 3231 3A30 3905", "BFC0 C0FC 2031 323A 3232 3A30 3906", "BFC0 C0FC 2031 323A 3233 3A30 3907", "BFC0 C0FC 2031 323A 3234 3A30 3908", "BFC0 C0FC 2031 323A 3235 3A30 3909", "BFC0 C0FC 2031 323A 3236 3A30 3910", "BFC0 C0FC 2031 323A 3237 3A30 3911", "BFC0 C0FC 2031 323A 3238 3A30 3912", "BFC0 C0FC 2031 323A 3239 3A30 3913", "BFC0 C0FC 2031 323A 3036 3A33 3214", "BFC0 C0FC 2031 323A 3037 3A33 3215", "BFC0 C0FC 2031 323A 3038 3A33 3216", "BFC0 C0FC 2031 323A 3038 3A33 3217", "BFC0 C0FC 2031 323A 3039 3A33 3218", "BFC0 C0FC 2031 323A 3039 3A35 3019", "BFC0 C0FC 2031 323A 3130 3A35 3020", "BFC0 C0FC 2031 323A 3131 3A35 3121", "BFC0 C8C4 2031 313A 3536 3A33 3222", "BFC0 C8C4 2031 313A 3537 3A33 3223", "BFC0 C8C4 2031 313A 3538 3A33 3224", "BFC0 C8C4 2031 313A 3539 3A33 3225", "BFC0 C0FC 2031 323A 3030 3A33 3226", "BFC0 C0FC 2031 323A 3031 3A33 3227", "BFC0 C0FC 2031 323A 3032 3A33 3228", "BFC0 C0FC 2031 323A 3033 3A33 3229", "BFC0 C0FC 2031 323A 3034 3A33 3230", "BFC0 C0FC 2031 323A 3035 3A33 3231", "BFC0 C0FC 2031 323A 3036 3A33 3232", "BFC0 C0FC 2031 323A 3037 3A33 3233", "BFC0 C0FC 2031 323A 3038 3A33 3234", "BFC0 C0FC 2033 3A34 373A 3031 0035 ", "BFC0 C0FC 2033 3A34 383A 3234 0036", "BFC0 C0FC 2033 3A34 393A 3132 0037", "BFC0 C0FC 2033 3A35 303A 3534 0038", "BFC0 C0FC 2033 3A35 313A 3231 0039 ", "BFC0 C0FC 2033 3A35 323A 3333 0040 ", "BFC0 C0FC 2033 3A35 333A 3030 0041", "BFC0 C0FC 2033 3A35 343A 3432 0042", "BFC0 C0FC 2033 3A35 353A 3431 0043", "BFC0 C0FC 2033 3A35 363A 3131 0044", "BFC0 C0FC 2033 3A35 373A 3239 0045", "BFC0 C0FC 2033 3A35 383A 3539 0046", "BFC0 C0FC 2033 3A35 393A 3533 0047", "BFC0 C0FC 2034 3A30 303A 3430 0048 "] ("출력 배열"), index=w142) -> (element=w141:string)
          n65 = Equal?(x=w141) -> (y=w140:string)  [unwired: 1 out]
        }
        frame Enabled {
        }
      }
      n66 = call "ip address.vi"() -> ("ip address"=w136:string)  [unwired: 11 in]
      "ip address" <- w136
      n67 = call <vilib>:"Space Constant.vi"() -> ("String"=w135:string)
      n68 = call <vilib>:"Space Constant.vi"() -> ("String"=w138:string)
      n69 = Concatenate Strings("serial number ", w138, w128, "의 IP는", w135, w136, w135, "입니다.") -> (w133:string)
      n70 = call "E-메일 보내기"("Message"=w133, "Subject"="ATC appliction customer IP , serial number ") -> ("error out"=w131:errorcluster)  [unwired: 9 in]
      n71 = call <vilib>:"Clear Errors.vi"("error in (no error)"=w131, "specific error code to clear (0: all)"=0) -> ()  [unwired: 4 in, 2 out]
    }
    frame #2 {
      n72 = while {
        stop <- FALSE stop-if-true
        n73 = while {
          stop <- FALSE stop-if-true
          n74 = flat-sequence {
            tunnel: [w338] -> w334
            tunnel: "콜사인" -> [w338]
            tunnel: "인사말" -> [w337]
            tunnel: w334 -> [w339]
            tunnel: [w339] -> w333
            tunnel: w333 -> [w340]
            tunnel: [w340] -> w332
            tunnel: w332 -> [w341]
            tunnel: [w341] -> w331
            tunnel: [w342] -> w330
            tunnel: w331 -> [w342]
            tunnel: w330 -> [w343]
            tunnel: [w343] -> w329
            tunnel: [w344] -> w328
            tunnel: w329 -> [w344]
            tunnel: w328 -> [w345]
            tunnel: [w345] -> w327
            tunnel: w327 -> [w346]
            tunnel: [w346] -> w326
            tunnel: w326 -> [w347]
            tunnel: [w347] -> w325
            tunnel: w325 -> [w348]
            tunnel: [w348] -> w324
            tunnel: w324 -> [w349]
            tunnel: [w349] -> w323
            tunnel: w323 -> [w350]
            tunnel: [w350] -> w322
            tunnel: w322 -> [w351]
            frame #0 {
              n75 = local write "인사말2"(w337) -> ()
              n76 = local write "인사말"(w337) -> ()
              n77 = local write "인사말 2"(w337) -> ()
              n78 = local write "인사4"(w337) -> ()
              n79 = local write "인사5"(w337) -> ()
              n80 = local write "인사3"(w337) -> ()
              n81 = local write "콜사인3"(w338) -> ()
              n82 = local write "콜사인2"(w338) -> ()
              n83 = local write "콜사인4"(w338) -> ()
              n84 = local write "콜사인"(w338) -> ()
            }
            frame #1 {
              n85 = local write "콜사인5"(w339) -> ()
              n86 = local write "콜사인6"(w339) -> ()
              n87 = local write "콜사인7"(w339) -> ()
              n88 = local write "콜사인8"(w339) -> ()
            }
            frame #2 {
              n89 = local write "콜사인10"(w340) -> ()
              n90 = local write "콜사인11"(w340) -> ()
              n91 = local write "콜사인9"(w340) -> ()
              n92 = local write "콜사인12"(w340) -> ()
              n93 = local write "콜사인13"(w340) -> ()
              n94 = local write "콜사인14"(w340) -> ()
            }
            frame #3 {
              n95 = local write "콜사인15"(w341) -> ()
              n96 = local write "콜사인16"(w341) -> ()
              n97 = local write "콜사인17"(w341) -> ()
              n98 = local write "콜사인18"(w341) -> ()
              n99 = local write "콜사인19"(w341) -> ()
              n100 = local write "콜사인20"(w341) -> ()
            }
            frame #4 {
              n101 = local write "콜사인21"(w342) -> ()
              n102 = local write "콜사인22"(w342) -> ()
              n103 = local write "콜사인23"(w342) -> ()
              n104 = local write "콜사인24"(w342) -> ()
              n105 = local write "콜사인25"(w342) -> ()
              n106 = local write "콜사인26"(w342) -> ()
            }
            frame #5 {
              n107 = local write "콜사인28"(w343) -> ()
              n108 = local write "콜사인29"(w343) -> ()
              n109 = local write "콜사인30"(w343) -> ()
              n110 = local write "콜사인31"(w343) -> ()
              n111 = local write "콜사인32"(w343) -> ()
            }
            frame #6 {
              n112 = local write "콜사인34 2"(w344) -> ()
              n113 = local write "콜사인33"(w344) -> ()
              n114 = local write "콜사인34"(w344) -> ()
              n115 = local write "콜사인53"(w344) -> ()
              n116 = local write "콜사인54"(w344) -> ()
              n117 = local write "콜사인55"(w344) -> ()
              n118 = local write "콜사인56"(w344) -> ()
            }
            frame #7 {
              n119 = local write "콜사인57"(w345) -> ()
              n120 = local write "콜사인58"(w345) -> ()
              n121 = local write "콜사인59"(w345) -> ()
              n122 = local write "콜사인35"(w345) -> ()
              n123 = local write "콜사인36"(w345) -> ()
              n124 = local write "콜사인37"(w345) -> ()
            }
            frame #8 {
              n125 = local write "콜사인39 2"(w346) -> ()
              n126 = local write "콜사인38"(w346) -> ()
              n127 = local write "콜사인39"(w346) -> ()
              n128 = local write "콜사인40"(w346) -> ()
              n129 = local write "콜사인41"(w346) -> ()
            }
            frame #9 {
              n130 = local write "콜사인38 2"(w347) -> ()
              n131 = local write "콜사인46"(w347) -> ()
              n132 = local write "콜사인47"(w347) -> ()
              n133 = local write "콜사인48"(w347) -> ()
              n134 = local write "콜사인49"(w347) -> ()
              n135 = local write "콜사인50"(w347) -> ()
              n136 = local write "콜사인51"(w347) -> ()
            }
            frame #10 {
              n137 = local write "콜사인60"(w348) -> ()
              n138 = local write "콜사인61"(w348) -> ()
              n139 = local write "콜사인62"(w348) -> ()
              n140 = local write "콜사인63"(w348) -> ()
              n141 = local write "콜사인64"(w348) -> ()
            }
            frame #11 {
              n142 = local write "콜사인65"(w349) -> ()
              n143 = local write "콜사인66"(w349) -> ()
              n144 = local write "콜사인67"(w349) -> ()
              n145 = local write "콜사인68"(w349) -> ()
            }
            frame #12 {
              n146 = local write "콜사인69"(w350) -> ()
              n147 = local write "콜사인69"(w350) -> ()
              n148 = local write "콜사인70"(w350) -> ()
            }
            frame #13 {
              n149 = local write "콜사인72"(w351) -> ()
              n150 = local write "콜사인71"(w351) -> ()
            }
          }
          n151 = flat-sequence {
            tunnel: "L활주로" -> [w354]
            tunnel: [w354] -> w336
            tunnel: w336 -> [w355]
            frame #0 {
              n152 = local write "L활주로3"(w354) -> ()
              n153 = local write "L활주로6"(w354) -> ()
              n154 = local write "L활주로"(w354) -> ()
              n155 = local write "L활주로"(w354) -> ()
              n156 = local write "L활주로"(w354) -> ()
              n157 = local write "L활주로"(w354) -> ()
            }
            frame #1 {
              n158 = local write "L활주로7"(w355) -> ()
              n159 = local write "L활주로"(w355) -> ()
              n160 = local write "L활주로"(w355) -> ()
              n161 = local write "L활주로"(w355) -> ()
            }
          }
          n162 = flat-sequence {
            tunnel: [w352] -> w335
            tunnel: "활주로1" -> [w352]
            tunnel: w335 -> [w353]
            frame #0 {
              n163 = local write "활주로1"(w352) -> ()
              n164 = local write "활주로2"(w352) -> ()
              n165 = local write "활주로3"(w352) -> ()
              n166 = local write "활주로4"(w352) -> ()
              n167 = local write "활주로5"(w352) -> ()
              n168 = local write "활주로6"(w352) -> ()
              n169 = local write "활주로7"(w352) -> ()
            }
            frame #1 {
              n170 = local write "활주로10"(w353) -> ()
              n171 = local write "활주로12"(w353) -> ()
              n172 = local write "활주로13"(w353) -> ()
              n173 = local write "활주로14"(w353) -> ()
              n174 = local write "활주로15"(w353) -> ()
              n175 = local write "활주로8"(w353) -> ()
              n176 = local write "활주로9"(w353) -> ()
            }
          }
          n177 = Wait (ms)(milliseconds to wait=u32 800 ("대기 시간(ms)")) -> ()  [unwired: 1 out]
        }
        n178 = while {
          stop <- FALSE stop-if-true
          # "출발공항의 바람"
          # "도착공항의 바람정보"
          n179 = local write "제한고도2"("제한고도") -> ()
          n180 = local write "ILS2"("ILS") -> ()
          n181 = local write "관제기관3"("T관제기관") -> ()
          n182 = local write "T관제기관"("T관제기관") -> ()
          n183 = local write "접속주파수2"("접속주파수") -> ()
          n184 = local write "ILS"("ILS") -> ()
          n185 = local write "제한고도"("제한고도") -> ()
          n186 = local write "관제기관"("T관제기관") -> ()
          n187 = local write "관제기관"("T관제기관") -> ()
          n188 = local write "관제기관"("T관제기관") -> ()
          n189 = local write "접속주파수"("접속주파수") -> ()
          n190 = local write "방향 2"("방향") -> ()
          n191 = local write "유도로 2"("유도로 2") -> ()
          n192 = local write "유도로"("유도로 2") -> ()
          n193 = local write "방향"("방향") -> ()
          n194 = local write "고도"("고도") -> ()
          n195 = local write "고도"("고도") -> ()
          n196 = local write "스콱번호"("스콱번호") -> ()
          n197 = local write "스콱번호2"("스콱번호") -> ()
          n198 = local write "T접속주파수2"("T접속주파수") -> ()
          n199 = local write "T접속주파수"("T접속주파수") -> ()
          n200 = local write "허가고도7 3"("허가고도 2") -> ()
          n201 = local write "허가고도7 2"("허가고도 2") -> ()
          n202 = local write "허가고도 2"("허가고도 2") -> ()
          n203 = local write "현재기압"("현재기압") -> ()
          n204 = local write "현재기압"("현재기압") -> ()
          n205 = local write "고도"("고도") -> ()
          n206 = local write "고도"("고도") -> ()
          n207 = local write "THEN2"("THEN") -> ()
          n208 = local write "G접속주파수2"("G접속주파수") -> ()
          n209 = local write "THEN"("THEN") -> ()
          n210 = local write "G접속주파수"("G접속주파수") -> ()
          n211 = local write "지점"("지점") -> ()
          n212 = local write "지점 2"("지점") -> ()
          n213 = local write "바람방향"("바람방향") -> ()
          n214 = local write "D접속주파수2"("D접속주파수") -> ()
          n215 = local write "D접속주파수"("D접속주파수") -> ()
          n216 = local write "T접속주파수"("T접속주파수") -> ()
          n217 = local write "T접속주파수"("T접속주파수") -> ()
          n218 = local write "A접속주파수2"("A접속주파수") -> ()
          n219 = local write "A접속주파수"("A접속주파수") -> ()
          n220 = local write "풍속"("풍속") -> ()
          n221 = local write "G접속주파수"("G접속주파수") -> ()
          n222 = local write "G접속주파수"("G접속주파수") -> ()
          n223 = local write "비행고도2"("비행고도") -> ()
          n224 = local write "비행고도3"("비행고도") -> ()
          n225 = local write "비행고도"("비행고도") -> ()
          n226 = local write "도착공항2"("도착공항") -> ()
          n227 = local write "도착공항3"("도착공항") -> ()
          n228 = local write "도착공항4"("도착공항") -> ()
          n229 = local write "도착공항5"("도착공항") -> ()
          n230 = local write "게이트번호2"("게이트번호") -> ()
          n231 = local write "게이트번호"("게이트번호") -> ()
          n232 = local write "도착공항"("도착공항") -> ()
          n233 = local write "SID&RadarVector. 2"("SID&RadarVector") -> ()
          n234 = local write "SID&RadarVector. 3"("SID&RadarVector") -> ()
          n235 = local write "SID&RadarVector"("SID&RadarVector") -> ()
          n236 = local write "현재기압2"("현재기압") -> ()
          n237 = local write "현재기압"("현재기압") -> ()
          n238 = local write "관제기관"("관제기관") -> ()
          n239 = local write "관제기관"("관제기관") -> ()
          n240 = Wait (ms)(milliseconds to wait=u32 800 ("대기 시간(ms)")) -> ()  [unwired: 1 out]
        }
        n241 = Wait (ms)(milliseconds to wait=u32 0 ("대기 시간(ms)")) -> ()  [unwired: 1 out]
        n242 = while {
          stop <- FALSE stop-if-true
          n243 = Wait (ms)(milliseconds to wait=u32 800 ("대기 시간(ms)")) -> ()  [unwired: 1 out]
          n244 = event shown="[7] \"정보8\": 마우스 커서 들어옴" {
            selector: _ -> [_ _ _ _ _ _ _ _ _]
            dyn-events: _ -> [_ _ _ _ _ _ _ _ _]
            timeout: 100 -> [_ _ _ _ _ _ _ _ _]
            event "정보1": Mouse Enter {
              n245 = event-data() -> ()  [unwired: 1 in, 4 out]
              n246 = call "사용자에게 메시지 디스플레이4"() -> ()  [unwired: 10 in, 2 out]
            }
            event "정보2": Mouse Enter {
              n247 = event-data() -> ()  [unwired: 1 in, 4 out]
              n248 = call "사용자에게 메시지 디스플레이5"() -> ()  [unwired: 10 in, 2 out]
            }
            event "정보3": Mouse Enter {
              n249 = event-data() -> ()  [unwired: 1 in, 4 out]
              n250 = call "사용자에게 메시지 디스플레이6"() -> ()  [unwired: 10 in, 2 out]
            }
            event "정보4": Mouse Enter {
              n251 = event-data() -> ()  [unwired: 1 in, 4 out]
              n252 = call "사용자에게 메시지 디스플레이7"() -> ()  [unwired: 10 in, 2 out]
            }
            event "정보5": Mouse Enter {
              n253 = event-data() -> ()  [unwired: 1 in, 4 out]
              n254 = call "사용자에게 메시지 디스플레이10"() -> ()  [unwired: 10 in, 2 out]
            }
            event "정보6": Mouse Enter {
              n255 = event-data() -> ()  [unwired: 1 in, 4 out]
              n256 = call "사용자에게 메시지 디스플레이8"() -> ()  [unwired: 10 in, 2 out]
            }
            event "정보7": Mouse Enter {
              n257 = event-data() -> ()  [unwired: 1 in, 4 out]
              n258 = call "사용자에게 메시지 디스플레이9"() -> ()  [unwired: 10 in, 2 out]
            }
            event "정보8": Mouse Enter {
              n259 = event-data() -> ()  [unwired: 1 in, 4 out]
              n260 = call "사용자에게 메시지 디스플레이3"() -> ()  [unwired: 10 in, 2 out]
            }
            event Timeout {
              n261 = event-data() -> ()  [unwired: 1 in, 3 out]
            }
          }
        }
        n262 = while {
          stop <- FALSE stop-if-true
          n263 = event shown="[7] \"도움말 8\": 마우스 다운" {
            selector: _ -> [_ _ _ _ _ _ _ _ _]
            dyn-events: _ -> [_ _ _ _ _ _ _ _ _]
            timeout: 10 -> [_ _ _ _ _ _ _ _ _]
            event "도움말": Mouse Down {
              w159 = 128  # call and forget
              n264 = event-data() -> ()  [unwired: 1 in, 8 out]
              n265 = vi-ref "popup.vi"() -> (w152:refnum<vi>)
              n266 = property class="VI"(reference=w152) -> (error out=w150:errorcluster, "Name"=w151:string)  [unwired: 1 in, 1 out]
              n267 = Open VI Reference(type specifier VI Refnum (for type only)=refnum<vi> refnum, vi path=w151, options=w159, error in (no error)=w150) -> (vi reference=w157:refnum<vi>, error out=w156:errorcluster)  [unwired: 2 in]
              n268 = call-by-ref "Start Asynchronous Call"(reference=w157, error in=w156) -> (reference out=w154:refnum<vi>, error out=w155:errorcluster)  [unwired: 12 in]
              n269 = Close Reference(reference=w154, error in (no error)=w155) -> (error out=w153:errorcluster)
              n270 = call <vilib>:"Simple Error Handler.vi"("error in (no error)"=w153) -> ()  [unwired: 4 in, 5 out]
            }
            event "도움말 2": Mouse Down {
              w169 = 128  # call and forget
              n271 = event-data() -> ()  [unwired: 1 in, 8 out]
              n272 = vi-ref "popup.vi"() -> (w162:refnum<vi>)
              n273 = property class="VI"(reference=w162) -> (error out=w160:errorcluster, "Name"=w161:string)  [unwired: 1 in, 1 out]
              n274 = Open VI Reference(type specifier VI Refnum (for type only)=refnum<vi> refnum, vi path=w161, options=w169, error in (no error)=w160) -> (vi reference=w167:refnum<vi>, error out=w166:errorcluster)  [unwired: 2 in]
              n275 = call-by-ref "Start Asynchronous Call"(reference=w167, error in=w166) -> (reference out=w164:refnum<vi>, error out=w165:errorcluster)  [unwired: 12 in]
              n276 = Close Reference(reference=w164, error in (no error)=w165) -> (error out=w163:errorcluster)
              n277 = call <vilib>:"Simple Error Handler.vi"("error in (no error)"=w163) -> ()  [unwired: 4 in, 5 out]
            }
            event "도움말 3": Mouse Down {
              w179 = 128  # call and forget
              n278 = event-data() -> ()  [unwired: 1 in, 8 out]
              n279 = vi-ref "popup.vi"() -> (w172:refnum<vi>)
              n280 = property class="VI"(reference=w172) -> (error out=w170:errorcluster, "Name"=w171:string)  [unwired: 1 in, 1 out]
              n281 = Open VI Reference(type specifier VI Refnum (for type only)=refnum<vi> refnum, vi path=w171, options=w179, error in (no error)=w170) -> (vi reference=w177:refnum<vi>, error out=w176:errorcluster)  [unwired: 2 in]
              n282 = call-by-ref "Start Asynchronous Call"(reference=w177, error in=w176) -> (reference out=w174:refnum<vi>, error out=w175:errorcluster)  [unwired: 12 in]
              n283 = Close Reference(reference=w174, error in (no error)=w175) -> (error out=w173:errorcluster)
              n284 = call <vilib>:"Simple Error Handler.vi"("error in (no error)"=w173) -> ()  [unwired: 4 in, 5 out]
            }
            event "도움말 4": Mouse Down {
              w189 = 128  # call and forget
              n285 = event-data() -> ()  [unwired: 1 in, 8 out]
              n286 = vi-ref "popup.vi"() -> (w182:refnum<vi>)
              n287 = property class="VI"(reference=w182) -> (error out=w180:errorcluster, "Name"=w181:string)  [unwired: 1 in, 1 out]
              n288 = Open VI Reference(type specifier VI Refnum (for type only)=refnum<vi> refnum, vi path=w181, options=w189, error in (no error)=w180) -> (vi reference=w187:refnum<vi>, error out=w186:errorcluster)  [unwired: 2 in]
              n289 = call-by-ref "Start Asynchronous Call"(reference=w187, error in=w186) -> (reference out=w184:refnum<vi>, error out=w185:errorcluster)  [unwired: 12 in]
              n290 = Close Reference(reference=w184, error in (no error)=w185) -> (error out=w183:errorcluster)
              n291 = call <vilib>:"Simple Error Handler.vi"("error in (no error)"=w183) -> ()  [unwired: 4 in, 5 out]
            }
            event "도움말 5": Mouse Down {
              w199 = 128  # call and forget
              n292 = event-data() -> ()  [unwired: 1 in, 8 out]
              n293 = vi-ref "popup.vi"() -> (w192:refnum<vi>)
              n294 = property class="VI"(reference=w192) -> (error out=w190:errorcluster, "Name"=w191:string)  [unwired: 1 in, 1 out]
              n295 = Open VI Reference(type specifier VI Refnum (for type only)=refnum<vi> refnum, vi path=w191, options=w199, error in (no error)=w190) -> (vi reference=w197:refnum<vi>, error out=w196:errorcluster)  [unwired: 2 in]
              n296 = call-by-ref "Start Asynchronous Call"(reference=w197, error in=w196) -> (reference out=w194:refnum<vi>, error out=w195:errorcluster)  [unwired: 12 in]
              n297 = Close Reference(reference=w194, error in (no error)=w195) -> (error out=w193:errorcluster)
              n298 = call <vilib>:"Simple Error Handler.vi"("error in (no error)"=w193) -> ()  [unwired: 4 in, 5 out]
            }
            event "도움말 6": Mouse Down {
              w209 = 128  # call and forget
              n299 = event-data() -> ()  [unwired: 1 in, 8 out]
              n300 = vi-ref "popup.vi"() -> (w202:refnum<vi>)
              n301 = property class="VI"(reference=w202) -> (error out=w200:errorcluster, "Name"=w201:string)  [unwired: 1 in, 1 out]
              n302 = Open VI Reference(type specifier VI Refnum (for type only)=refnum<vi> refnum, vi path=w201, options=w209, error in (no error)=w200) -> (vi reference=w207:refnum<vi>, error out=w206:errorcluster)  [unwired: 2 in]
              n303 = call-by-ref "Start Asynchronous Call"(reference=w207, error in=w206) -> (reference out=w204:refnum<vi>, error out=w205:errorcluster)  [unwired: 12 in]
              n304 = Close Reference(reference=w204, error in (no error)=w205) -> (error out=w203:errorcluster)
              n305 = call <vilib>:"Simple Error Handler.vi"("error in (no error)"=w203) -> ()  [unwired: 4 in, 5 out]
            }
            event "도움말 7": Mouse Down {
              w219 = 128  # call and forget
              n306 = event-data() -> ()  [unwired: 1 in, 8 out]
              n307 = vi-ref "popup.vi"() -> (w212:refnum<vi>)
              n308 = property class="VI"(reference=w212) -> (error out=w210:errorcluster, "Name"=w211:string)  [unwired: 1 in, 1 out]
              n309 = Open VI Reference(type specifier VI Refnum (for type only)=refnum<vi> refnum, vi path=w211, options=w219, error in (no error)=w210) -> (vi reference=w217:refnum<vi>, error out=w216:errorcluster)  [unwired: 2 in]
              n310 = call-by-ref "Start Asynchronous Call"(reference=w217, error in=w216) -> (reference out=w214:refnum<vi>, error out=w215:errorcluster)  [unwired: 12 in]
              n311 = Close Reference(reference=w214, error in (no error)=w215) -> (error out=w213:errorcluster)
              n312 = call <vilib>:"Simple Error Handler.vi"("error in (no error)"=w213) -> ()  [unwired: 4 in, 5 out]
            }
            event "도움말 8": Mouse Down {
              w225 = T3 11 items=["사용자 홈"=0, "사용자 데스크탑"=1, "사용자 문서"=2, "사용자 어플리케이션 데이터"=3, "사용자 환경"=4, "사용자 임시"=5, "퍼블릭 문서"=6, "퍼블릭 어플리케이션 데이터"=7, "퍼블릭 환경"=8, "퍼블릭 캐시"=13, "시스템 코어 라이브러리"=9, "시스템 설치된 라이브러리"=10, "어플리케이션 파일"=11, "부팅 볼륨 루트"=12] ("system directory type")
              w220 = 256  # call and forget
              n313 = event-data() -> ()  [unwired: 1 in, 8 out]
              n314 = call <vilib>:"Get System Directory.vi"("system directory type"=w225) -> ("system directory"=w224:path)  [unwired: 10 in]
              n315 = Build Path(base path=w224, name or relative path="popup.vi" ("이름 또는 상대 경로")) -> (appended path=w222:path)
              n316 = Open VI Reference(type specifier VI Refnum (for type only)=refnum<vi> refnum, vi path=w222, options=w220) -> (vi reference=w228:refnum<vi>, error out=w229:errorcluster)  [unwired: 3 in]
              n317 = call-by-ref "비동기화 호출 기다림"(reference=w228, error in=w229) -> (reference out=w226:refnum<vi>, error out=w227:errorcluster)  [unwired: 12 in]
              n318 = call-by-ref "Start Asynchronous Call"(reference=w226, error in=w227) -> (reference out=w230:refnum<vi>, error out=w231:errorcluster)  [unwired: 12 in]
              n319 = Close Reference(reference=w230, error in (no error)=w231) -> ()  [unwired: 1 out]
            }
            event Timeout {
              n320 = event-data() -> ()  [unwired: 1 in, 3 out]
            }
          }
        }
        n321 = while {
          stop <- FALSE stop-if-true
          n322 = local write "G관제기관"("G관제기관") -> ()
          n323 = local write "관제기관3 2"("G관제기관") -> ()
          n324 = local write "관제기관2"("G관제기관") -> ()
          n325 = local write "관제기관"("G관제기관") -> ()
          n326 = local write "관제기관"("G관제기관") -> ()
          n327 = local write "관제기관4"("G관제기관") -> ()
          n328 = case shown="참" "?" {
            frame False {
            }
            frame True {
              w379 = T3 2 items=["사용자 홈"=0, "사용자 데스크탑"=1, "사용자 문서"=2, "사용자 어플리케이션 데이터"=3, "사용자 환경"=4, "사용자 임시"=5, "퍼블릭 문서"=6, "퍼블릭 어플리케이션 데이터"=7, "퍼블릭 환경"=8, "퍼블릭 캐시"=13, "시스템 코어 라이브러리"=9, "시스템 설치된 라이브러리"=10, "어플리케이션 파일"=11, "부팅 볼륨 루트"=12] ("system directory type")
              n329 = call <vilib>:"Get System Directory.vi"("create directory if not found? (F)"=TRUE, "system directory type"=w379) -> ("system directory"=w381:path)  [unwired: 9 in]
              n330 = Build Path(base path=w381, name or relative path="ATC app output.txt" ("이름 또는 상대 경로")) -> (appended path=w378:path)
              n331 = Open/Create/Replace File(file path (use dialog)=w378) -> (refnum out=w382:refnum<file>, error out=w383:errorcluster)  [unwired: 5 in, 1 out]
              n332 = Read from Text File(file (use dialog)=w382, error in=w383) -> (refnum out=w384:refnum<file>, text=w390:string, error out=w385:errorcluster)  [unwired: 2 in, 1 out]
              n333 = One Button Dialog(message="문서를 불러왔습니다." ("메시지")) -> ()  [unwired: 1 in, 1 out]
              n334 = Match Pattern "Clearance Delivery~Ground"(string=w390, regular expression="Clearance Delivery" ("정규식")) -> (after substring=w387:string)  [unwired: 1 in, 3 out]
              n335 = Close File(refnum=w384, error in=w385) -> ()  [unwired: 2 out]
              n336 = Match Pattern "Clearance Delivery~Ground"(string=w387, regular expression="Ground" ("정규식")) -> (before substring=w392:string, after substring=w391:string)  [unwired: 1 in, 2 out]
              n337 = call <vilib>:"Trim Whitespace.vi"("string"=w392) -> ("trimmed string"=w376:string)  [unwired: 1 in]
              n338 = Match Pattern "Tower(Departure) ~Departure"(string=w391, regular expression="Tower(Departure)" ("정규식")) -> (before substring=w393:string, after substring=w396:string)  [unwired: 1 in, 2 out]
              n339 = local write "메모"(w376) -> ()
              n340 = call <vilib>:"Trim Whitespace.vi"("string"=w393) -> ("trimmed string"=w375:string)  [unwired: 1 in]
              n341 = Match Pattern "Tower(Departure) ~Departure"(string=w396, regular expression="Departure" ("정규식")) -> (before substring=w395:string, after substring=w402:string)  [unwired: 1 in, 2 out]
              n342 = local write "메모2"(w375) -> ()
              n343 = call <vilib>:"Trim Whitespace.vi"("string"=w395) -> ("trimmed string"=w374:string)  [unwired: 1 in]
              n344 = Match Pattern "control~Approach"(string=w402, regular expression="control" ("정규식")) -> (before substring=w400:string, after substring=w398:string)  [unwired: 1 in, 2 out]
              n345 = local write "메모3"(w374) -> ()
              n346 = call <vilib>:"Trim Whitespace.vi"("string"=w400) -> ("trimmed string"=w373:string)  [unwired: 1 in]
              n347 = Match Pattern "control~Approach"(string=w398, regular expression="Approach" ("정규식")) -> (before substring=w401:string, after substring=w370:string)  [unwired: 1 in, 2 out]
              n348 = Match Pattern "Tower(Arrival)~Ground(Arrival)"(string=w370, regular expression="Tower(Arrival)" ("정규식")) -> (before substring=w368:string, after substring=w366:string)  [unwired: 1 in, 2 out]
              n349 = local write "메모 4"(w373) -> ()
              n350 = call <vilib>:"Trim Whitespace.vi"("string"=w401) -> ("trimmed string"=w372:string)  [unwired: 1 in]
              n351 = Match Pattern "Tower(Arrival)~Ground(Arrival)"(string=w366, regular expression="Ground(Arrival)" ("정규식")) -> (before substring=w365:string, after substring=w364:string)  [unwired: 1 in, 2 out]
              n352 = local write "메모6"(w368) -> ()
              n353 = local write "메모5"(w372) -> ()
              n354 = local write "메모7"(w365) -> ()
              n355 = local write "메모8"(w364) -> ()
            }
          }
          n356 = local write "관제기관5"("G관제기관") -> ()
          n357 = local write "관제기관"("G관제기관") -> ()
          n358 = local write "관제기관"("G관제기관") -> ()
          n359 = local write "출발공항2"("출발공항") -> ()
          n360 = local write "출발공항"("출발공항") -> ()
          n361 = local write "C활주로3"("C활주로") -> ()
          n362 = local write "C활주로2"("C활주로") -> ()
          n363 = local write "C활주로"("C활주로") -> ()
          n364 = Wait (ms)(milliseconds to wait=u32 800 ("대기 시간(ms)")) -> ()  [unwired: 1 out]
          n365 = local write "허가고도6 3"("허가고도") -> ()
          n366 = local write "허가고도6 2"("허가고도") -> ()
          n367 = local write "허가고도4"("허가고도") -> ()
          n368 = local write "허가고도5"("허가고도") -> ()
          n369 = local write "허가고도6"("허가고도") -> ()
          n370 = local write "허가고도7"("허가고도") -> ()
          n371 = local write "허가고도"("허가고도") -> ()
          n372 = case shown="참" "?" {
            frame False {
            }
            frame True {
              w406 = "\r"
              w414 = "\r"
              w417 = "\r"
              w422 = "\r"
              w431 = T3 2 items=["사용자 홈"=0, "사용자 데스크탑"=1, "사용자 문서"=2, "사용자 어플리케이션 데이터"=3, "사용자 환경"=4, "사용자 임시"=5, "퍼블릭 문서"=6, "퍼블릭 어플리케이션 데이터"=7, "퍼블릭 환경"=8, "퍼블릭 캐시"=13, "시스템 코어 라이브러리"=9, "시스템 설치된 라이브러리"=10, "어플리케이션 파일"=11, "부팅 볼륨 루트"=12] ("system directory type")
              n373 = call <vilib>:"Get System Directory.vi"("create directory if not found? (F)"=TRUE, "system directory type"=w431) -> ("system directory"=w436:path)  [unwired: 9 in]
              n374 = Build Path(base path=w436, name or relative path="ATC app output.txt" ("이름 또는 상대 경로")) -> (appended path=w434:path)
              n375 = One Button Dialog(message="문서 폴더에 저장되었습니다." ("메시지")) -> ()  [unwired: 1 in, 1 out]
              n376 = Concatenate Strings("Clearance Delivery", "\r", "메모", "\r", "Ground", "\r", "메모2", w422, "Tower(Departure)", w422, "메모3", "\r", "Departure", w417, "메모 4", w417, "control", w414, "메모5", w414, "Approach", w414, "메모6", w406, "Tower(Arrival)", w406, "메모7", w406, "Ground(Arrival)", "\r", "메모8") -> (w413:string)
              n377 = Write to Text File(file (use dialog)=w434, text=w413) -> (refnum out=w433:refnum<file>, error out=w432:errorcluster)  [unwired: 2 in, 1 out]
              n378 = Close File(refnum=w433, error in=w432) -> ()  [unwired: 2 out]
            }
          }
        }
        n379 = while {
          stop <- FALSE stop-if-true
          n380 = event shown="[0] 키 다운" {
            selector: _ -> [_ _]
            dyn-events: _ -> [_ _]
            timeout: 0 -> [_ _]
            event Key Down {
              n381 = event-data() -> ("Char"=w236:i16)  [unwired: 1 in, 9 out]
              n382 = Equal?(x=w236, y=i16 43) -> (x = y?=w237:bool)
              n383 = case shown="참" w237 {
                frame False {
                }
                frame True {
                  w242 = T3 2 items=["사용자 홈"=0, "사용자 데스크탑"=1, "사용자 문서"=2, "사용자 어플리케이션 데이터"=3, "사용자 환경"=4, "사용자 임시"=5, "퍼블릭 문서"=6, "퍼블릭 어플리케이션 데이터"=7, "퍼블릭 환경"=8, "퍼블릭 캐시"=13, "시스템 코어 라이브러리"=9, "시스템 설치된 라이브러리"=10, "어플리케이션 파일"=11, "부팅 볼륨 루트"=12] ("system directory type")
                  n384 = call <vilib>:"Get System Directory.vi"("create directory if not found? (F)"=TRUE, "system directory type"=w242) -> ("system directory"=w241:path)  [unwired: 9 in]
                  n385 = Build Path(base path=w241, name or relative path="ATC app output.txt" ("이름 또는 상대 경로")) -> (appended path=w265:path)
                  n386 = Open/Create/Replace File(file path (use dialog)=w265) -> (refnum out=w264:refnum<file>, error out=w263:errorcluster)  [unwired: 5 in, 1 out]
                  n387 = Read from Text File(file (use dialog)=w264, error in=w263) -> (refnum out=w262:refnum<file>, text=w256:string, error out=w261:errorcluster)  [unwired: 2 in, 1 out]
                  n388 = Match Pattern "Clearance Delivery~Ground"(string=w256, regular expression="Clearance Delivery" ("정규식")) -> (after substring=w259:string)  [unwired: 1 in, 3 out]
                  n389 = Close File(refnum=w262, error in=w261) -> ()  [unwired: 2 out]
                  n390 = Match Pattern "Clearance Delivery~Ground"(string=w259, regular expression="Ground" ("정규식")) -> (before substring=w254:string, after substring=w255:string)  [unwired: 1 in, 2 out]
                  n391 = One Button Dialog(message="문서를 불러왔습니다." ("메시지")) -> ()  [unwired: 1 in, 1 out]
                  n392 = call <vilib>:"Trim Whitespace.vi"("string"=w254) -> ("trimmed string"=w266:string)  [unwired: 1 in]
                  n393 = Match Pattern "Tower(Departure) ~Departure"(string=w255, regular expression="Tower(Departure)" ("정규식")) -> (before substring=w253:string, after substring=w250:string)  [unwired: 1 in, 2 out]
                  n394 = local write "메모"(w266) -> ()
                  n395 = call <vilib>:"Trim Whitespace.vi"("string"=w253) -> ("trimmed string"=w267:string)  [unwired: 1 in]
                  n396 = Match Pattern "Tower(Departure) ~Departure"(string=w250, regular expression="Departure" ("정규식")) -> (before substring=w251:string, after substring=w244:string)  [unwired: 1 in, 2 out]
                  n397 = local write "메모2"(w267) -> ()
                  n398 = call <vilib>:"Trim Whitespace.vi"("string"=w251) -> ("trimmed string"=w268:string)  [unwired: 1 in]
                  n399 = Match Pattern "control~Approach"(string=w244, regular expression="control" ("정규식")) -> (before substring=w246:string, after substring=w248:string)  [unwired: 1 in, 2 out]
                  n400 = local write "메모3"(w268) -> ()
                  n401 = call <vilib>:"Trim Whitespace.vi"("string"=w246) -> ("trimmed string"=w269:string)  [unwired: 1 in]
                  n402 = Match Pattern "control~Approach"(string=w248, regular expression="Approach" ("정규식")) -> (before substring=w245:string, after substring=w272:string)  [unwired: 1 in, 2 out]
                  n403 = Match Pattern "Tower(Arrival)~Ground(Arrival)"(string=w272, regular expression="Tower(Arrival)" ("정규식")) -> (before substring=w274:string, after substring=w276:string)  [unwired: 1 in, 2 out]
                  n404 = local write "메모 4"(w269) -> ()
                  n405 = call <vilib>:"Trim Whitespace.vi"("string"=w245) -> ("trimmed string"=w270:string)  [unwired: 1 in]
                  n406 = Match Pattern "Tower(Arrival)~Ground(Arrival)"(string=w276, regular expression="Ground(Arrival)" ("정규식")) -> (before substring=w277:string, after substring=w278:string)  [unwired: 1 in, 2 out]
                  n407 = local write "메모6"(w274) -> ()
                  n408 = local write "메모5"(w270) -> ()
                  n409 = local write "메모7"(w277) -> ()
                  n410 = local write "메모8"(w278) -> ()
                }
              }
              n411 = Equal?(x=w236, y=i16 45) -> (x = y?=w239:bool)
              n412 = case shown="참" w239 {
                frame False {
                }
                frame True {
                  w282 = "\r"
                  w295 = "\r"
                  w297 = "\r"
                  w300 = "\r"
                  w307 = T3 2 items=["사용자 홈"=0, "사용자 데스크탑"=1, "사용자 문서"=2, "사용자 어플리케이션 데이터"=3, "사용자 환경"=4, "사용자 임시"=5, "퍼블릭 문서"=6, "퍼블릭 어플리케이션 데이터"=7, "퍼블릭 환경"=8, "퍼블릭 캐시"=13, "시스템 코어 라이브러리"=9, "시스템 설치된 라이브러리"=10, "어플리케이션 파일"=11, "부팅 볼륨 루트"=12] ("system directory type")
                  n413 = local read "메모6"() -> (w285:string)
                  n414 = local read "메모5"() -> (w286:string)
                  n415 = local read "메모 4"() -> (w287:string)
                  n416 = local read "메모7"() -> (w283:string)
                  n417 = local read "메모2"() -> (w289:string)
                  n418 = local read "메모3"() -> (w288:string)
                  n419 = local read "메모"() -> (w290:string)
                  n420 = local read "메모8"() -> (w279:string)
                  n421 = One Button Dialog(message="문서 폴더에 저장되었습니다." ("메시지")) -> ()  [unwired: 1 in, 1 out]
                  n422 = Concatenate Strings("Clearance Delivery", "\r", w290, "\r", "Ground", "\r", w289, w300, "Tower(Departure)", w300, w288, "\r", "Departure", w297, w287, w297, "control", w295, w286, w295, "Approach", w295, w285, w282, "Tower(Arrival)", w282, w283, w282, " Ground(Arrival)", "\r", w279) -> (w294:string)
                  n423 = call <vilib>:"Get System Directory.vi"("create directory if not found? (F)"=TRUE, "system directory type"=w307) -> ("system directory"=w312:path)  [unwired: 9 in]
                  n424 = Build Path(base path=w312, name or relative path="ATC app output.txt" ("이름 또는 상대 경로")) -> (appended path=w310:path)
                  n425 = Write to Text File(file (use dialog)=w310, text=w294) -> (refnum out=w309:refnum<file>, error out=w308:errorcluster)  [unwired: 2 in, 1 out]
                  n426 = Close File(refnum=w309, error in=w308) -> ()  [unwired: 2 out]
                }
              }
            }
            event Timeout {
              n427 = event-data() -> ()  [unwired: 1 in, 3 out]
            }
          }
          n428 = Wait (ms)(milliseconds to wait=u32 800 ("대기 시간(ms)")) -> ()  [unwired: 1 out]
        }
      }
    }
  }
